vi "move to field and wait.vi"(6 "Time Target":dbl[unit]=0.2 caption="Time Target (s)", 8 "error in (no error)":errorcluster, 9 "tolerance":dbl[unit]=1e-05, 10 "Setpoint":dbl[unit], 11 "VISA session":refnum<visa-resource-name>) -> (0 "error out":errorcluster, 3 "dup VISA session":refnum<visa-resource-name>)   [LabVIEW 2017]
panel:
  out "Setpoint ramping?\n(first half of requirement)":bool
  out "Field reading":dbl[unit]
  out "Elapsed Time\n(second half of requirement)":dbl[unit] caption="Elapsed Time (s)"
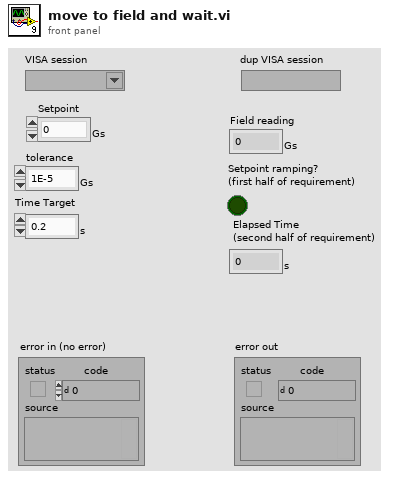
[diagram p1: front panel]
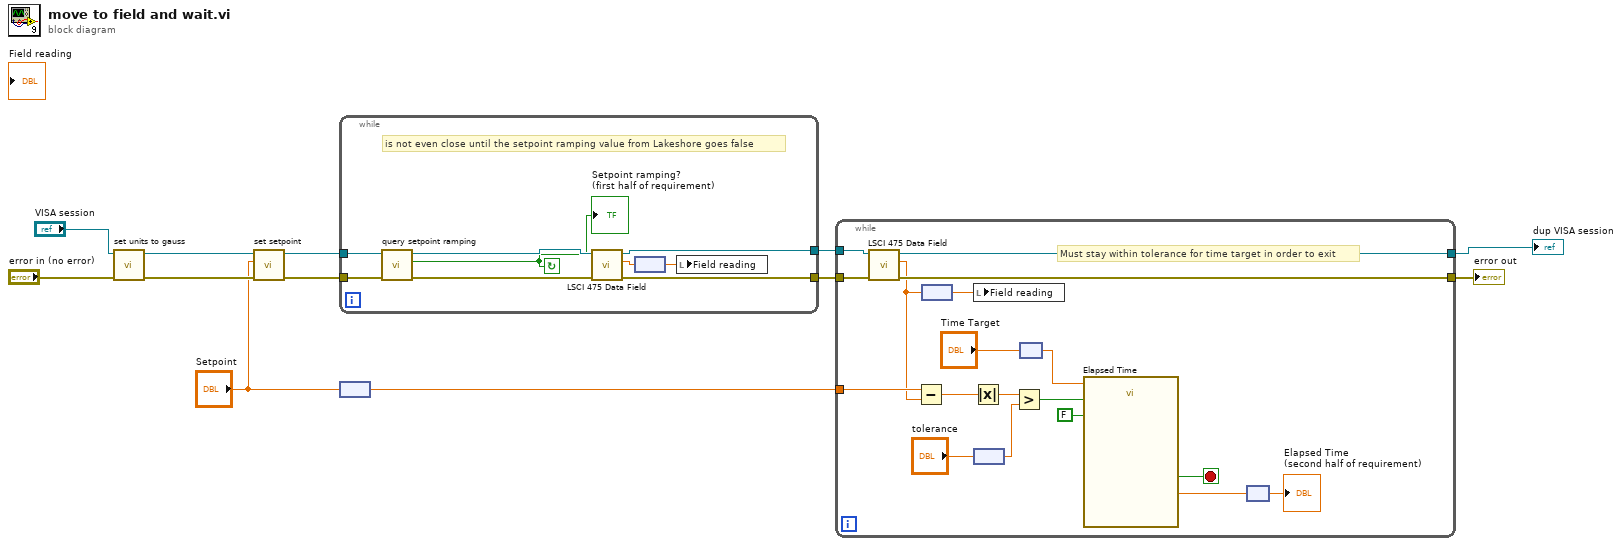
[diagram p0: block diagram]
diagram:
  n1 = call "set units to gauss.vi"("VISA session"="VISA session", "error in (no error)"="error in (no error)") -> ("dup VISA session"=w3:refnum<visa-resource-name>, "error out"=w4:errorcluster)  [unwired: 7 in]
  n2 = call "set setpoint.vi"("error in (no error)"=w4, "Setpoint"="Setpoint", "VISA session"=w3) -> ("error out"=w11:errorcluster, "dup VISA session"=w12:refnum<visa-resource-name>)  [unwired: 7 in]
  n3 = while {
    tunnel: [w18] -> w10
    tunnel: w12 -> [w20]
    tunnel: [w16] -> w8
    tunnel: w11 -> [w21]
    stop <- w15 continue-if-true
    # "is not even close until the setpoint ramping value from Lakeshore goes false"
    n4 = call "query setpoint ramping.vi"("error in (no error)"=w21, "VISA session"=w20) -> ("error out"=w17:errorcluster, "Setpoint Ramping?"=w15:bool, "dup VISA session"=w19:refnum<visa-resource-name>)  [unwired: 7 in]
    "Setpoint ramping?\n(first half of requirement)" <- w15
    n5 = call "LSCI 475 Data Field.vi"("error in (no error)"=w17, "VISA session"=w19) -> ("error out"=w16:errorcluster, "Field Reading"=w14:dbl, "dup VISA session"=w18:refnum<visa-resource-name>)  [unwired: 7 in]
    n6 = node(w14) -> (w13:dbl[unit])
    n7 = local write "Field reading"(w13) -> ()
  }
  n8 = node("Setpoint") -> (w1:dbl)
  n9 = while {
    tunnel: w1 -> [w38]
    tunnel: w10 -> [w37]
    tunnel: [w36] -> w9
    tunnel: [w35] -> w7
    tunnel: w8 -> [w34]
    stop <- w32 stop-if-true
    # "Must stay within tolerance for time target in order to exit"
    n10 = call "LSCI 475 Data Field.vi"("error in (no error)"=w34, "VISA session"=w37) -> ("error out"=w35:errorcluster, "Field Reading"=w29:dbl, "dup VISA session"=w36:refnum<visa-resource-name>)  [unwired: 7 in]
    n11 = Subtract(x=w38, y=w29) -> (x-y=w39:dbl)
    n12 = node(w29) -> (w28:dbl[unit])
    n13 = Absolute Value(x=w39) -> (abs(x)=w33:dbl)
    n14 = local write "Field reading"(w28) -> ()
    n15 = node("tolerance") -> (w26:dbl)
    n16 = Greater?(x=w33, y=w26) -> (0:w31:bool)
    n17 = node("Time Target") -> (w24:dbl)
    n18 = call "Elapsed Time"("Time Target (s)"=w24, "Reset"=w31, "Auto Reset"=FALSE) -> ("Elapsed Time (s)"=w23:dbl, "Time has Elapsed"=w32:bool)  [unwired: 9 in, 6 out]
    n19 = node(w23) -> (→"Elapsed Time\n(second half of requirement)":dbl[unit])
  }
  "dup VISA session" <- w9
  "error out" <- w7
